vi "Create_filter_points.vi"(2 "Precision":string, 4 "Non-Blank Rows":bool[](array[boolean]), 6 "notSelectors?":bool, 7 "Index":i32, 8 "Channel to Filter On":i32, 9 "Tolerance":dbl=1.0 format="%.2f", 10 "Filter Bins 1":i32[](array[numeric]), 11 "Ch Values In":string[][](array[string])) -> (0 "Unchanged?":bool, 1 "Accept array":bool[][](array[boolean]), 3 "Filter Bins Out":i32[](array[numeric]), 5 "Bin Names":string[](array[string]))   [LabVIEW 2022 SP3]
uses:
  Results_plotter_Global.vi
panel:
  in  "Filter Info":T1={"Filter Bins"=[], "Channel to Filter On"=0, "Bin Matches"=[], "Number of Rows"=0, "Bin Names"=[], "Tolerance"=1.0, "Indicies for all bins"=[]} {"Tolerance" format="%.2f"}
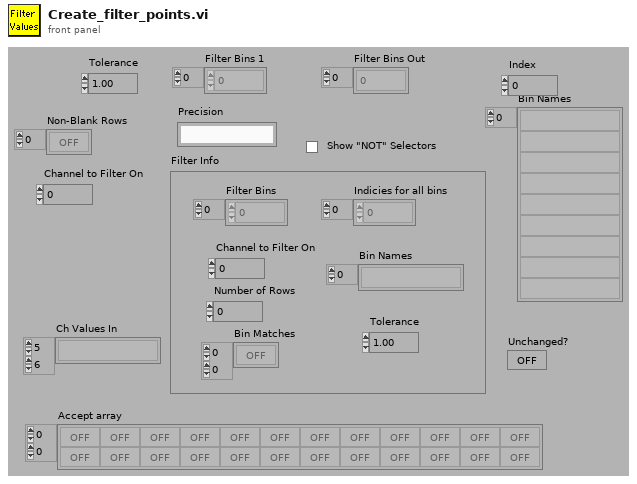
[diagram p1: front panel]
types:
  T1 = cluster{"Filter Bins":i32[], "Channel to Filter On":i32, "Bin Matches":bool[][], "Number of Rows":i32, "Bin Names":string[], "Tolerance":dbl, "Indicies for all bins":i32[]}
  T2 = cluster{"Filter Bins":i32[], "Channel to Filter On":i32, "Bin Matches":bool[][], "Number of Rows":i32, "Bin Names":string[], "Tolerance":dbl, "Indicies for all bins":i32[]}[]
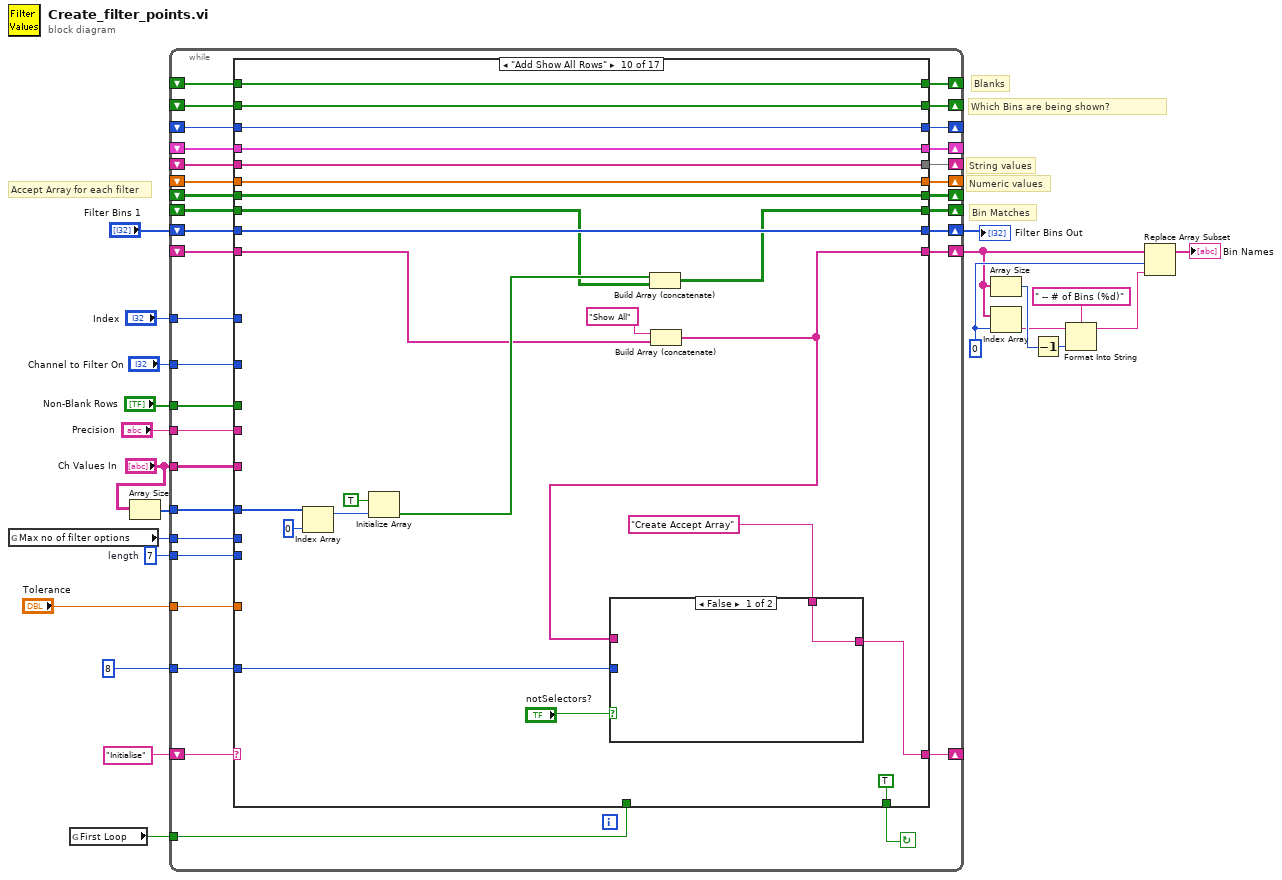
[diagram p0: block diagram]
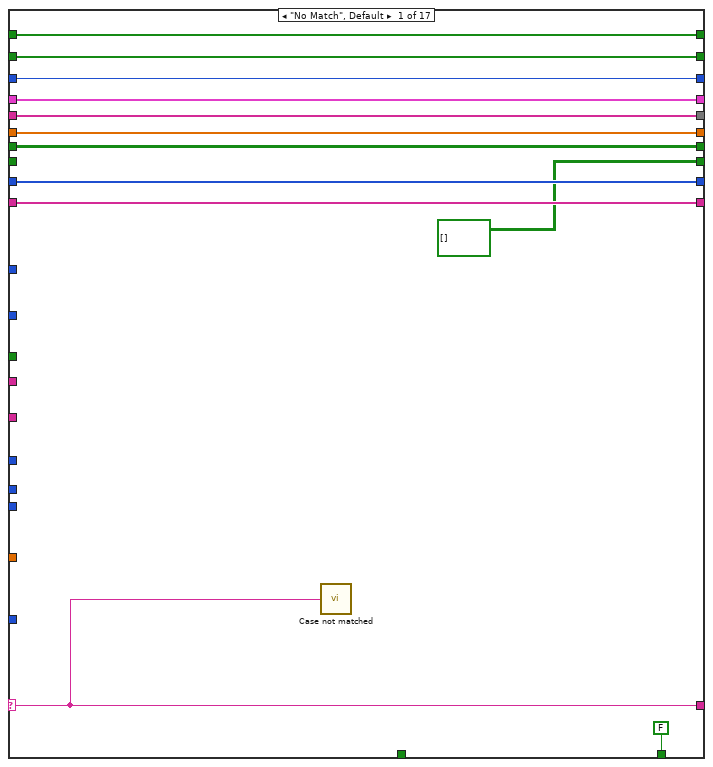
[diagram p2: hidden frame]
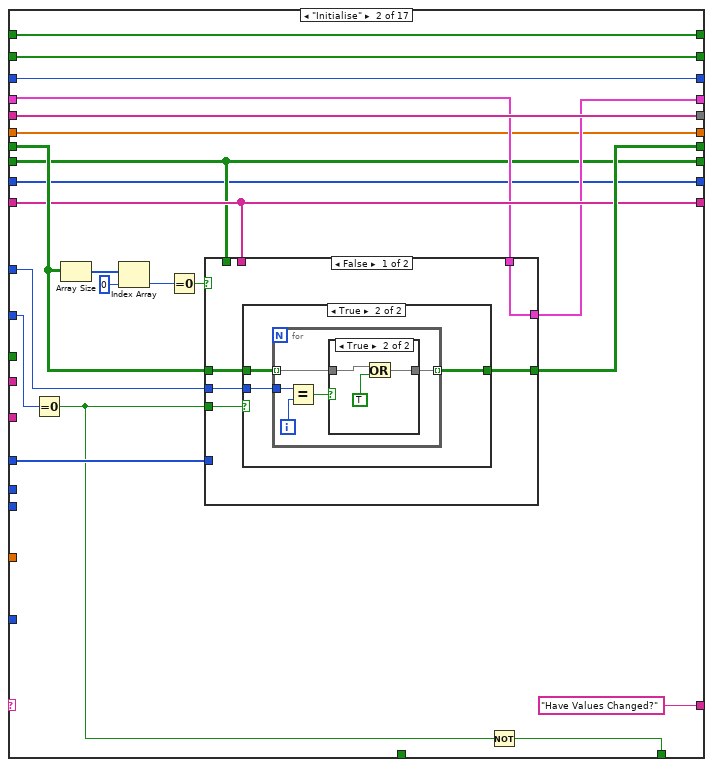
[diagram p3: hidden frame]
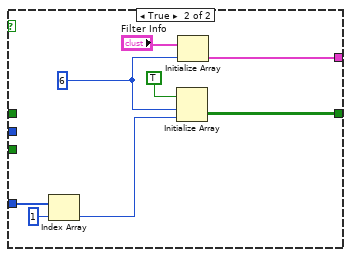
[diagram p6: hidden frame]
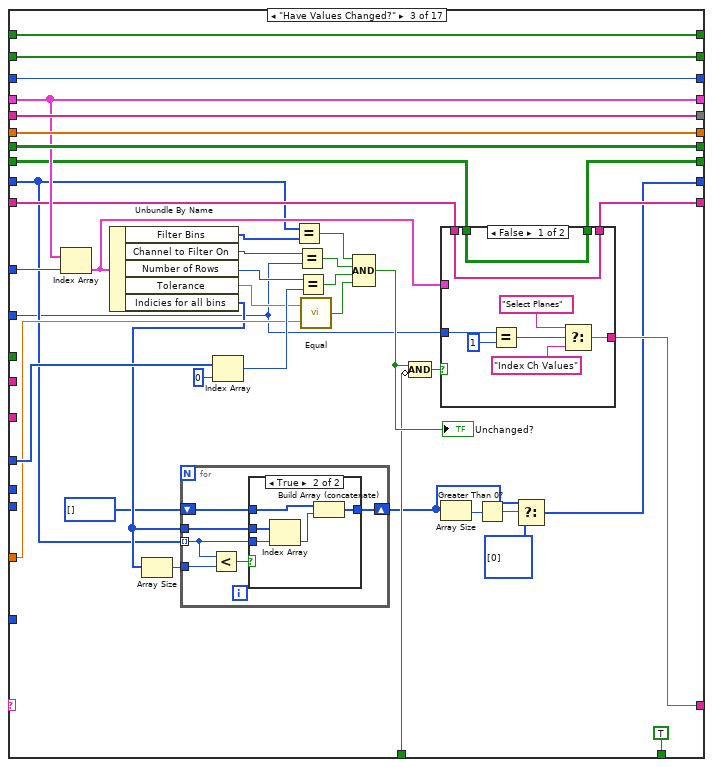
[diagram p7: hidden frame]
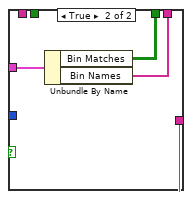
[diagram p9: hidden frame]
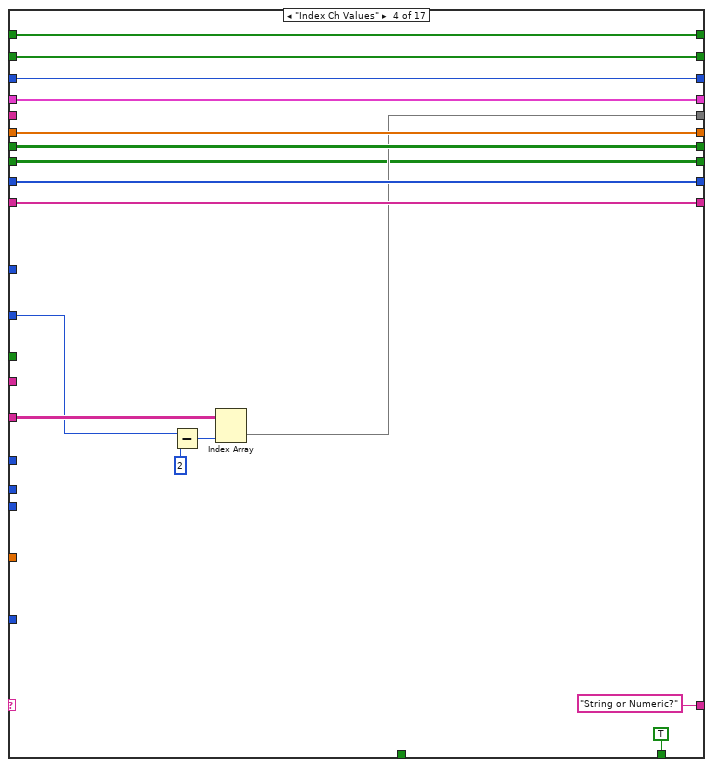
[diagram p10: hidden frame]
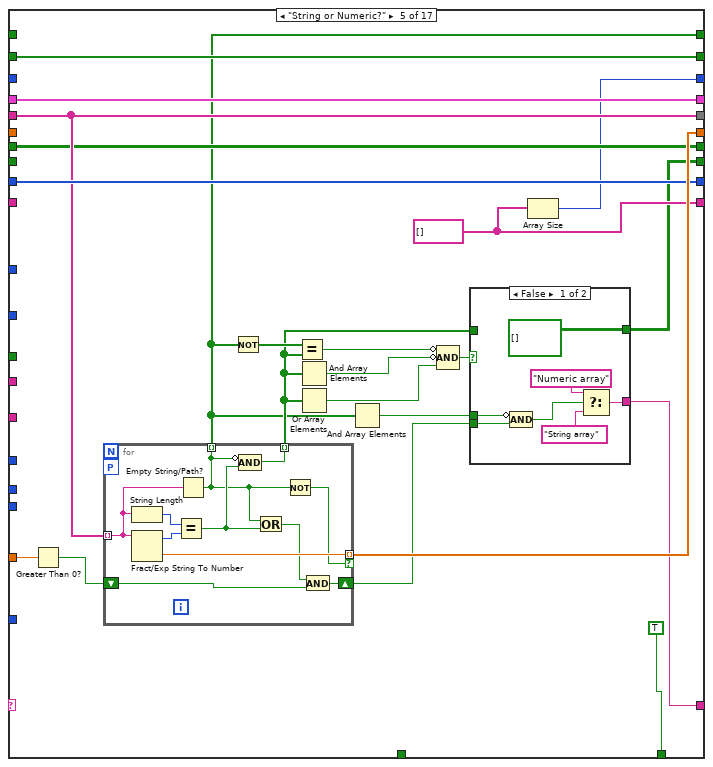
[diagram p11: hidden frame]
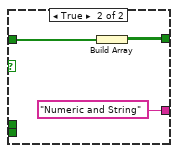
[diagram p12: hidden frame]
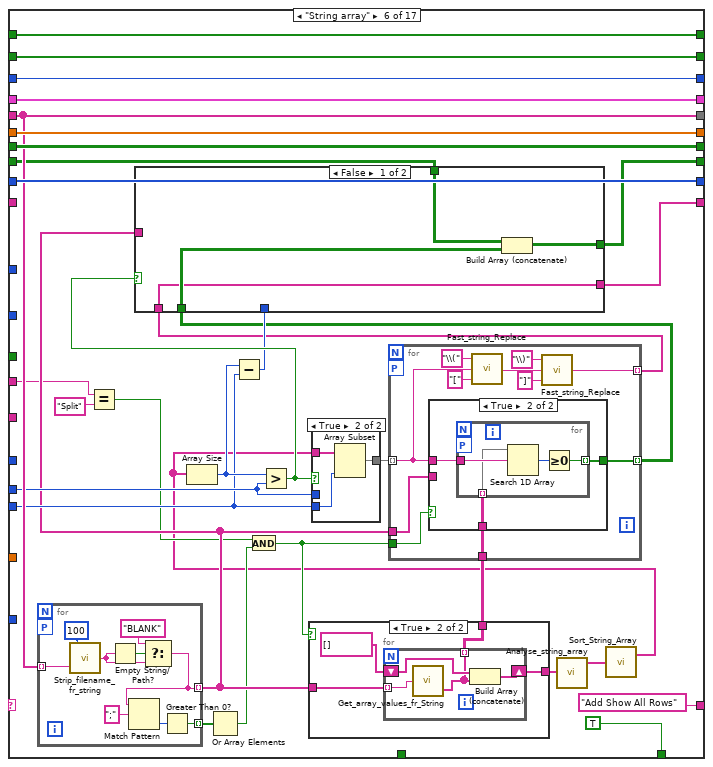
[diagram p13: hidden frame]
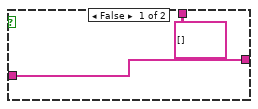
[diagram p14: hidden frame]
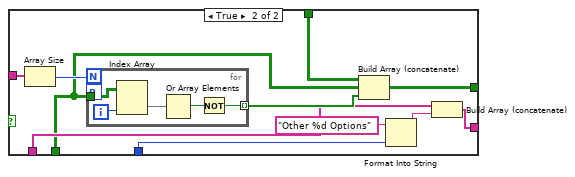
[diagram p15: hidden frame]
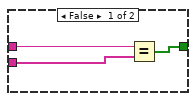
[diagram p17: hidden frame]
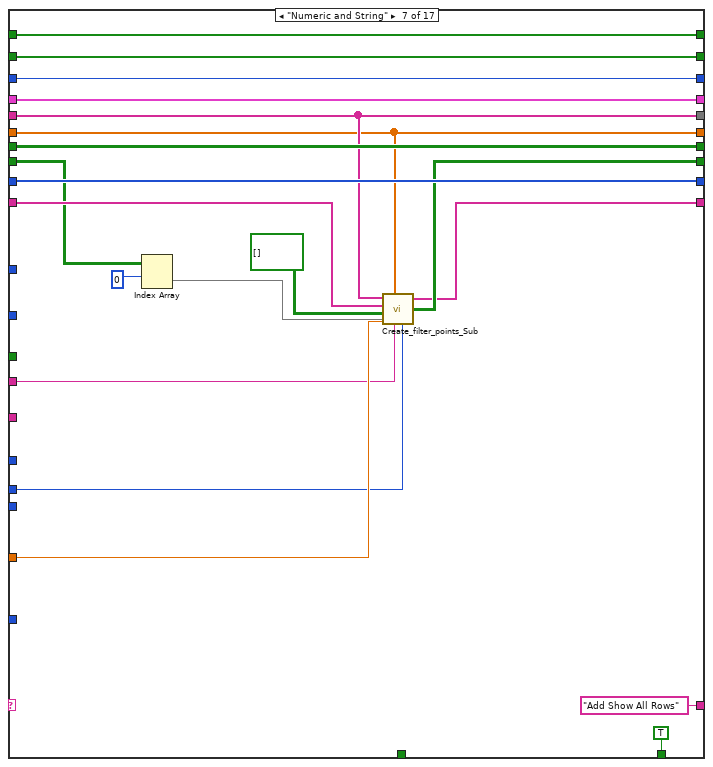
[diagram p18: hidden frame]
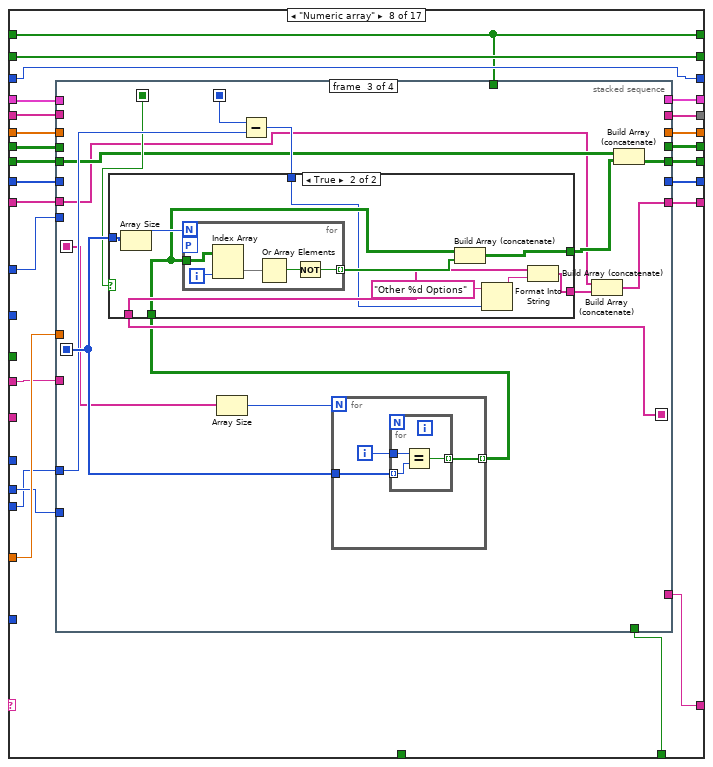
[diagram p19: hidden frame]
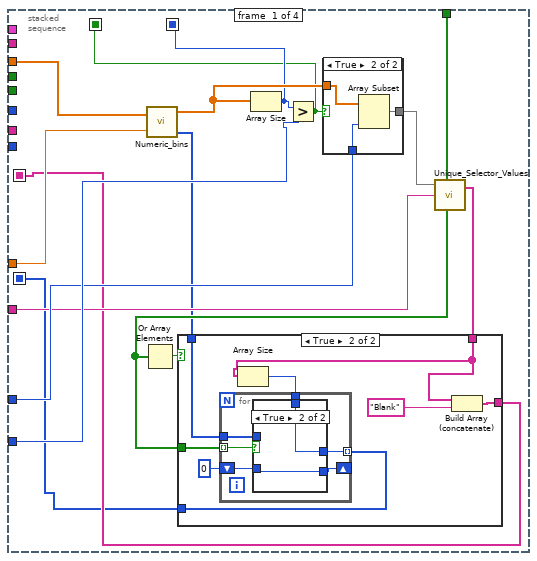
[diagram p20: hidden frame]
diagram:
  w7 = 0 ("index")
  w12 = 7  # length
  # "Blanks"
  # "Which Bins are being shown?"
  # "Accept Array for each filter"
  # "String values"
  # "Bin Matches"
  # "Numeric values"
  n1 = global read "Results_plotter_Global.vi" "Max no of filter options"() -> (w13:i32)
  n2 = global read "Results_plotter_Global.vi" "First Loop"() -> (w16:bool)
  n3 = Array Size(array="Ch Values In") -> (size(s)=w18:i32[])
  n4 = while {
    tunnel: "Non-Blank Rows" -> [w38]
    tunnel: w18 -> [w39]
    tunnel: "Channel to Filter On" -> [w41]
    shift-left: _ -> [w43]
    shift-right: [w42] -> _
    shift-left: _ -> [w44]
    shift-right: [w40] -> _
    shift-left: "Filter Bins 1" -> [w46]
    shift-right: [w45] -> w10
    tunnel: "Index" -> [w48]
    shift-left: _ -> [w47]
    shift-right: [w49] -> w6
    shift-left: _ -> [w35]
    shift-right: [w32] -> _
    shift-left: _ -> [w53]
    shift-right: [w52] -> _
    shift-left: _ -> [w50]
    shift-right: [w55] -> _
    shift-left: "Initialise" -> [w51]
    shift-right: [w25] -> _
    tunnel: "Ch Values In" -> [w56]
    tunnel: w16 -> [w37]
    tunnel: "Tolerance" -> [w36]
    shift-right: [w34] -> _
    shift-left: _ -> [w33]
    tunnel: "Precision" -> [w31]
    shift-right: [w30] -> _
    shift-left: _ -> [w29]
    tunnel: w13 -> [w28]
    tunnel: w12 -> [w27]
    tunnel: 8 ("y") -> [w26]
    shift-right: [w24] -> _
    shift-left: _ -> [w23]
    stop <- w54 continue-if-true
    n5 = case shown="\"Add Show All Rows\"" w51 {
      selector: w51 -> [w57 _ _ _ _ _ _ _ _ _ _ _ _ _ _ _ _]
      tunnel: w56 -> [_ _ _ w188 _ _ _ _ w501 _ _ _ _ _ _ _ _]
      tunnel: [w67 w76 w155 w194 w218 w270 w343 w376 w521 w704 w731 w752 w795 w848 w867 w895 w935] -> w55
      tunnel: [w57 "Have Values Changed?" w140 "String or Numeric?" w204 "Add Show All Rows" "Add Show All Rows" w378 w523 w689 "Create Accept Array" "Add Number of hits" "Relocate Selector?" w837 "Stop invalid selections" "Update shift Register" "End"] -> w25
      tunnel: [FALSE w79 TRUE TRUE TRUE TRUE TRUE w379 w524 TRUE TRUE TRUE TRUE TRUE TRUE TRUE FALSE] -> w54
      tunnel: w53 -> [w66 w86 w154 w193 w212 w267 w352 w374 w519 w703 w730 w747 w792 w846 w866 w894 w934]
      tunnel: [w66 w87 w154 w193 w212 w267 w352 w373 w518 w703 w730 w746 w792 w846 w866 w894 w934] -> w52
      tunnel: w50 -> [w67 w76 w155 w194 _ w270 w343 w375 w520 w704 w731 w752 w795 w848 w867 w895 w935]
      tunnel: [w65 w82 w139 w191 w200 w257 w344 w377 w522 w691 w718 w750 w790 w845 w864 w892 w914] -> w49
      tunnel: w48 -> [_ w85 w152 _ _ _ _ w369 w514 _ _ w749 w796 w835 w863 _ w932]
      tunnel: w35 -> [_ w77 w141 w187 _ w260 w346 w371 w516 w697 w723 w740 w784 w847 w859 w890 w925]
      tunnel: w47 -> [w65 w82 w138 w191 _ _ w347 w363 w508 w696 w719 w750 w787 w845 w864 w892 w917]
      tunnel: w46 -> [w62 w75 w119 w192 w216 w266 w351 w370 w515 w707 w734 w744 w799 w850 w857 w888 w912]
      tunnel: [w62 w75 w120 w192 w216 w266 w351 w364 w509 w707 w734 w744 w799 w850 w852 w884 w911] -> w45
      tunnel: w44 -> [w64 w84 w153 _ w214 w264 w350 w368 w513 w705 w732 w753 w797 w849 w865 w893 w933]
      tunnel: w43 -> [w63 w80 w151 w190 w215 w268 w353 w366 w511 w706 w733 w754 w798 w843 w855 w887 w931]
      tunnel: [w63 w81 w151 w190 w215 w268 w353 w365 w510 w706 w733 w754 w798 w843 w855 w887 w930] -> w42
      tunnel: w41 -> [_ w83 w118 w183 _ _ _ _ _ _ _ _ _ _ _ _ w924]
      tunnel: [w64 w84 w153 w189 w214 w264 w350 w367 w512 w705 w732 w753 w797 w849 w865 w893 w933] -> w40
      tunnel: [bool[][] [] w77 w128 w187 w199 w258 w345 w372 w517 w688 w722 w740 w784 w847 w859 w890 w925] -> w32
      tunnel: w39 -> [_ w74 w150 _ _ _ _ _ _ w701 _ _ _ _ _ _ w929]
      tunnel: w38 -> [_ _ _ _ _ _ _ _ _ _ _ w743 w794 _ _ _ _]
      tunnel: w37 -> [_ _ w132 _ _ _ _ _ _ _ _ _ _ _ _ _ _]
      tunnel: w36 -> [_ _ w131 _ w203 _ w349 w362 w507 _ _ _ _ _ _ _ w920]
      tunnel: [w61 w71 w130 w186 w202 w265 w342 w357 w502 w693 w727 w742 w791 w834 w854 w886 w919] -> w34
      tunnel: w33 -> [w61 w71 w130 w186 _ w265 w342 w357 w502 w693 w727 w742 w791 w834 w854 w886 w919]
      tunnel: w31 -> [_ _ _ _ _ w246 w341 w361 w506 _ _ _ _ _ _ _ _]
      tunnel: [w59 w70 w129 w185 w201 w263 w340 w360 w505 w692 w717 w741 w789 w833 w853 w885 w918] -> w30
      tunnel: w29 -> [w59 w70 w129 w185 w201 w263 w340 w360 w505 w692 w717 w741 _ w833 w853 w885 w918]
      tunnel: w28 -> [_ _ _ _ _ w261 w339 w359 w504 _ _ _ w776 _ _ _ _]
      tunnel: w27 -> [_ _ _ _ _ w255 _ w358 w503 _ _ _ _ _ _ _ _]
      tunnel: w26 -> [_ _ _ _ _ _ _ _ _ w687 _ _ w778 _ _ _ _]
      tunnel: [w58 w69 w117 w181 w197 w240 w336 w356 w498 w686 w716 w739 w775 w832 w851 w883 w910] -> w24
      tunnel: w23 -> [w58 w69 w117 w181 _ w240 w336 w356 w498 w686 w716 w739 w775 w832 w851 w883 w910]
      frame "No Match", Default {
        n6 = call "Case not matched.vi"("Case Name not Matched"=w57) -> ()
      }
      frame "Initialise" {
        n7 = Equal To 0?(x=w83) -> (x = 0?=w73:bool)
        n8 = Array Size(array=w86) -> (size(s)=w90:i32[])
        n9 = Index Array(array=w90, index=0 ("Index")) -> (element=w88:i32)
        n10 = Equal To 0?(x=w88) -> (x = 0?=w72:bool)
        n11 = case shown="False" w72 {
          tunnel: [w95 w115] -> w87
          tunnel: w86 -> [w94 _]
          tunnel: w85 -> [w93 _]
          tunnel: w73 -> [w92 _]
          tunnel: w82 -> [_ _]
          tunnel: [w91 w113] -> w81
          tunnel: w80 -> [w91 _]
          tunnel: w77 -> [_ _]
          tunnel: w74 -> [_ w110]
          frame False {
            n12 = case shown="True" w92 {
              tunnel: [w96 w98] -> w95
              tunnel: w94 -> [w96 w97]
              tunnel: w93 -> [_ w99]
              frame False {
              }
              frame True {
                n13 = for {
                  tunnel: w99 -> [w104]
                  tunnel: [w101] -> w98 mode=indexing
                  tunnel: w97 -> [w100] mode=indexing
                  i -> [w103]
                  n14 = Equal?(x=w104, y=w103) -> (x = y?=w102:bool)
                  n15 = case shown="True" w102 {
                    tunnel: [w105 w106] -> w101
                    tunnel: w100 -> [w105 w107]
                    frame False {
                    }
                    frame True {
                      n16 = Or(x=w107, y=TRUE) -> (x .or. y?=w106:bool[])
                    }
                  }
                }
              }
            }
          }
          frame True {
            w114 = 6 ("Dimension Size")
            n17 = Index Array(array=w110, index=1 ("Index")) -> (element=w111:i32)
            n18 = Initialize Array(TRUE, w114, w111) -> (w115:bool[][])
            n19 = Initialize Array("Filter Info", w114) -> (w113:T2)
          }
        }
        n20 = Not(x=w73) -> (.not. x?=w79:bool)
      }
      frame "Have Values Changed?" {
        n21 = Index Array(array=w151, index=w152) -> (element=w142:T1)
        n22 = Unbundle By Name(w142) -> ("Filter Bins"=w137:i32[], "Channel to Filter On"=w148:i32, "Number of Rows"=w147:i32, "Tolerance"=w134:dbl, "Indicies for all bins"=w127:i32[])
        n23 = Array Size(array=w127) -> (size(s)=w126:i32)
        n24 = for {
          tunnel: w119 -> [w160] mode=indexing
          tunnel: w127 -> [w162]
          tunnel: w126 -> [w161]
          shift-right: [w158] -> w122
          shift-left: i32[] [] -> [w157]
          n25 = Less?(x=w160, y=w161) -> (x < y?=w159:bool)
          n26 = case shown="True" w159 {
            tunnel: w162 -> [_ w168]
            tunnel: w160 -> [_ w167]
            tunnel: [w163 w165] -> w158
            tunnel: w157 -> [w163 w164]
            frame False {
            }
            frame True {
              n27 = Index Array(array=w168, index=w167) -> (element=w166:i32)
              n28 = Build Array (concatenate)(w164, w166) -> (w165:i32[])
            }
          }
        }
        n29 = Index Array(array=w150, index=0 ("Index")) -> (element=w146:i32)
        n30 = Equal?(x=w119, y=w137) -> (x = y?=w145:bool)
        n31 = Equal?(x=w148, y=w118) -> (x = y?=w144:bool)
        n32 = Equal?(x=w147, y=w146) -> (x = y?=w143:bool)
        n33 = call "Equal.vi"("Input2"=w131, "Input1"=w134) -> ("Equal?"=w133:bool)
        n34 = Compound Arithmetic op=AND(w145, w144, w143, w133) -> (w135:bool)
        "Unchanged?" <- w135
        n35 = Compound Arithmetic op=AND(w135, invert w132) -> (w136:bool)
        n36 = case shown="False" w136 {
          tunnel: w142 -> [_ w180]
          tunnel: [w175 w178] -> w128
          tunnel: w141 -> [w175 _]
          tunnel: [w170 "Create Accept Array"] -> w140
          tunnel: [w176 w179] -> w139
          tunnel: w138 -> [w176 _]
          tunnel: w118 -> [w174 _]
          frame False {
            n37 = Equal?(x=w174, y=1) -> (x = y?=w172:bool)
            n38 = Select(t="Select Planes", s=w172, f="Index Ch Values") -> (s? t:f=w170:string)
          }
          frame True {
            n39 = Unbundle By Name(w180) -> ("Bin Matches"=w178:bool[][], "Bin Names"=w179:string[])
          }
        }
        n40 = Array Size(array=w122) -> (size(s)=w124:i32)
        n41 = Greater Than 0?(x=w124) -> (x > 0?=w123:bool)
        n42 = Select(t=w122, s=w123, f=i32[] [0]) -> (s? t:f=w120:i32[])
      }
      frame "Index Ch Values" {
        n43 = Subtract(x=w183, y=2) -> (x-y=w182:i32)
        n44 = Index Array(array=w188, index (col)=w182) -> (element=w189:string[])  [unwired: 1 in]
      }
      frame "String or Numeric?" {
        w200 = string[] []
        n45 = Greater Than 0?(x=w203) -> (x > 0?=w217:bool)
        n46 = for {
          tunnel: w214 -> [w235] mode=indexing
          shift-right: [w238] -> w205
          shift-left: w217 -> [w239]
          tunnel: [w232] -> w218 mode=indexing if=w230
          tunnel: [w229] -> w197 mode=indexing
          tunnel: [w233] -> w198 mode=indexing
          workers-P: _ -> [_]
          n47 = String Length(string=w235) -> (length=w236:i32)
          n48 = Fract/Exp String To Number(string=w235) -> (offset past number=w237:i32, number=w232:dbl)  [unwired: 3 out]
          n49 = Equal?(x=w236, y=w237) -> (x = y?=w234:bool)
          n50 = Empty String/Path?(string/path=w235) -> (empty?=w229:bool)
          n51 = Compound Arithmetic op=AND(invert w229, w234) -> (w233:bool)
          n52 = Or(x=w229, y=w234) -> (x .or. y?=w231:bool)
          n53 = Not(x=w229) -> (.not. x?=w230:bool)
          n54 = And(x=w231, y=w239) -> (x .and. y?=w238:bool)
        }
        n55 = Not(x=w197) -> (.not. x?=w207:bool[])
        n56 = Equal?(x=w207, y=w198) -> (x = y?=w208:bool)
        n57 = And Array Elements(Boolean array=w198) -> (logical AND=w211:bool)
        n58 = Or Array Elements(Boolean array=w198) -> (logical OR=w210:bool)
        n59 = And Array Elements(Boolean array=w197) -> (logical AND=w206:bool)
        n60 = Compound Arithmetic op=AND(invert w208, invert w211, w210) -> (w209:bool)
        n61 = case shown="False" w209 {
          tunnel: w206 -> [w225 _]
          tunnel: w205 -> [w224 _]
          tunnel: [w220 "Numeric and String"] -> w204
          tunnel: [bool[][] [] w226] -> w199
          tunnel: w198 -> [_ w227]
          frame False {
            n62 = Compound Arithmetic op=AND(invert w225, w224) -> (w221:bool)
            n63 = Select(t="Numeric array", s=w221, f="String array") -> (s? t:f=w220:string)
          }
          frame True {
            n64 = Build Array(w227) -> (w226:bool[][])
          }
        }
        n65 = Array Size(array=w200) -> (size(s)=w202:i32)
      }
      frame "String array" {
        n66 = for {
          tunnel: w264 -> [w314] mode=indexing
          tunnel: [w306] -> w249 mode=indexing
          tunnel: [w310] -> w251 mode=indexing
          workers-P: _ -> [_]
          n67 = call "Strip_filename_fr_string.vi"("Input String"=w314, "y"=100) -> ("Output String"=w307:string)
          n68 = Empty String/Path?(string/path=w307) -> (empty?=w309:bool)
          n69 = Select(t="BLANK", s=w309, f=w307) -> (s? t:f=w306:string)
          n70 = Match Pattern(string=w306, regular expression=";") -> (offset past match=w311:i32)  [unwired: 4 out]
          n71 = Greater Than 0?(x=w311) -> (x > 0?=w310:bool)
        }
        n72 = Equal?(x=w246, y="Split") -> (x = y?=w244:bool)
        n73 = Or Array Elements(Boolean array=w251) -> (logical OR=w245:bool)
        n74 = And(x=w244, y=w245) -> (x .and. y?=w243:bool)
        n75 = case shown="True" w243 {
          tunnel: [w273 w276] -> w250
          tunnel: w249 -> [w273 w275]
          tunnel: [string[][] [] ("String array") w274] -> w248
          frame False {
          }
          frame True {
            n76 = for {
              shift-right: [w281] -> w276
              shift-left: string[] [] -> [w280]
              tunnel: w275 -> [w279] mode=indexing
              tunnel: [w278] -> w274 mode=indexing
              n77 = call "Get_array_values_fr_String.vi"("String Value"=w279) -> ("String array"=w278:string[])  [unwired: 1 out]
              n78 = Build Array (concatenate)(w280, w278) -> (w281:string[])
            }
          }
        }
        n79 = call "Analyse_string_array.vi"("String array"=w250) -> ("Unique strings"=w242:string[])  [unwired: 2 out]
        n80 = call "Sort_String_Array.vi"("Unsorted String"=w242) -> ("Sorted String"=w241:string[])  [unwired: 1 out]
        n81 = Array Size(array=w241) -> (size(s)=w256:i32)
        n82 = Subtract(x=w256, y=w255) -> (x-y=w254:i32)
        n83 = Greater?(x=w256, y=w261) -> (0:w259:bool)
        n84 = case shown="True" w259 {
          tunnel: w241 -> [w302 w305]
          tunnel: w261 -> [_ _]
          tunnel: [w302 w304] -> w262
          tunnel: w255 -> [_ w303]
          frame False {
          }
          frame True {
            n85 = Array Subset(array=w305, length=w303) -> (w304:string[])  [unwired: 1 in]
          }
        }
        n86 = for {
          tunnel: w249 -> [w320]
          tunnel: w262 -> [w319] mode=indexing
          tunnel: [w315] -> w253 mode=indexing
          tunnel: [w318] -> w252 mode=indexing
          tunnel: w243 -> [w317]
          tunnel: w248 -> [w316]
          workers-P: _ -> [_]
          n87 = case shown="True" w317 {
            tunnel: w320 -> [w328 _]
            tunnel: w319 -> [w327 w331]
            tunnel: [w326 w330] -> w318
            tunnel: w316 -> [_ w329]
            frame False {
              n88 = Equal?(x=w327, y=w328) -> (x = y?=w326:bool[])
            }
            frame True {
              n89 = for {
                tunnel: w331 -> [w335]
                tunnel: [w333] -> w330 mode=indexing
                tunnel: w329 -> [w332] mode=indexing
                workers-P: _ -> [_]
                n90 = Search 1D Array(1D array=w332, element=w335) -> (index of element=w334:i32)  [unwired: 1 out]
                n91 = Greater Or Equal To 0?(x=w334) -> (x >= 0?=w333:bool)
              }
            }
          }
          n92 = call "Fast_string_Replace.vi"("Replace match with:"="[", "Input String"=w319, "regular expression"="\\(") -> ("Output String"=w321:string)  [unwired: 2 out]
          n93 = call "Fast_string_Replace.vi"("Replace match with:"="]", "Input String"=w321, "regular expression"="\\)") -> ("Output String"=w315:string)  [unwired: 2 out]
        }
        n94 = case shown="False" w259 {
          tunnel: w253 -> [w283 w293]
          tunnel: w260 -> [w285 w296]
          tunnel: w252 -> [w284 w286]
          tunnel: [w282 w294] -> w258
          tunnel: [w283 w292] -> w257
          tunnel: w249 -> [_ w291]
          tunnel: w254 -> [_ w289]
          frame False {
            n95 = Build Array (concatenate)(w285, w284) -> (w282:bool[][])
          }
          frame True {
            n96 = Array Size(array=w291) -> (size(s)=w290:i32)
            n97 = for {
              N: w290 -> [_]
              tunnel: w286 -> [w301]
              tunnel: [w297] -> w295 mode=indexing
              workers-P: _ -> [_]
              i -> [w300]
              n98 = Index Array(array=w301, index (col)=w300) -> (element=w299:bool[])  [unwired: 1 in]
              n99 = Or Array Elements(Boolean array=w299) -> (logical OR=w298:bool)
              n100 = Not(x=w298) -> (.not. x?=w297:bool)
            }
            n101 = Build Array (concatenate)(w296, w286, w295) -> (w294:bool[][])
            n102 = Format Into String(format string="Other %d Options", w289) -> (resulting string=w287:string)  [unwired: 2 in, 1 out]
            n103 = Build Array (concatenate)(w293, w287) -> (w292:string[])
          }
        }
      }
      frame "Numeric and String" {
        n104 = Index Array(array=w346, index (row)=0) -> (element=w348:bool[])  [unwired: 1 in]
        n105 = call "Create_filter_points_Sub.vi"("Numeric Value?"=w348, "No of filter options"=w339, "Precision"=w341, "Tolerance"=w349, "Bin Matches in"=bool[][] [] ("Bin Matches"), "Numeric Array"=w343, "Bin Names In"=w347, "String Array"=w350) -> ("Bin Matches"=w345:bool[][], "Bin Names"=w344:string[])  [unwired: 1 out]
      }
      frame "Numeric array" {
        n106 = stacked-sequence {
          seq-local: [w381 _ _ _] -> [_ _ w466 _]
          seq-local: [_ w422 _ _] -> [_ _ w467 _]
          seq-local: [w389 _ _ _] -> [_ _ w465 _]
          seq-local: [w388 _ _ _] -> [_ _ w462 _]
          seq-local: [w383 _ _ _] -> [_ w421 w453 _]
          tunnel: w362 -> [w393 _ _ _]
          tunnel: [_ _ _ w493] -> w376
          tunnel: w375 -> [w394 _ _ w493]
          tunnel: w374 -> [_ _ _ w492]
          tunnel: [_ _ _ w492] -> w373
          tunnel: [_ _ w459 _] -> w372
          tunnel: w371 -> [_ _ w458 _]
          tunnel: w370 -> [_ _ _ w491]
          tunnel: [_ _ _ w491] -> w364
          tunnel: [_ _ _ TRUE] -> w379
          tunnel: [_ _ _ "Add Show All Rows"] -> w378
          tunnel: [_ _ w456 _] -> w377
          tunnel: w369 -> [_ _ _ _]
          tunnel: w368 -> [_ _ _ w495]
          tunnel: [_ _ _ w495] -> w367
          tunnel: w366 -> [_ _ _ w494]
          tunnel: [_ _ _ w494] -> w365
          tunnel: w363 -> [_ _ w455 _]
          tunnel: w361 -> [w386 _ _ _]
          tunnel: w359 -> [w391 _ _ _]
          tunnel: w358 -> [w390 _ w464 _]
          tunnel: w356 -> [w382 _ _ _]
          frame #0 {
            n107 = Or Array Elements(Boolean array=w382) -> (logical OR=w385:bool)
            n108 = call "Numeric_bins.vi"("Values"=w394, "Tolerance"=w393) -> ("Bin Centres"=w392:dbl[], "Bin Index"=w380:i32[])  [unwired: 1 out]
            n109 = Array Size(array=w392) -> (size(s)=w389:i32)
            n110 = Greater?(x=w389, y=w391) -> (0:w388:bool)
            n111 = case shown="True" w388 {
              tunnel: w392 -> [w417 w420]
              tunnel: [w417 w419] -> w387
              tunnel: w390 -> [_ w418]
              frame False {
              }
              frame True {
                n112 = Array Subset(array=w420, length=w418) -> (w419:dbl[])  [unwired: 1 in]
              }
            }
            n113 = call "Unique_Selector_Values.vi"("Precision"=w386, "Bin Centres"=w387) -> ("Bin Strings"=w384:string[])  [unwired: 1 in, 1 out]
            n114 = case shown="True" w385 {
              tunnel: w384 -> [w396 w402]
              tunnel: [w396 w403] -> w383
              tunnel: w382 -> [_ w401]
              tunnel: [w395 w400] -> w381
              tunnel: w380 -> [w395 w397]
              frame False {
              }
              frame True {
                n115 = Array Size(array=w402) -> (size(s)=w399:i32)
                n116 = for {
                  shift-right: [w406] -> _
                  shift-left: 0 -> [w407]
                  tunnel: w401 -> [w410] mode=indexing
                  tunnel: [w409] -> w400 mode=indexing
                  tunnel: w399 -> [w408]
                  tunnel: w397 -> [w405]
                  n117 = case shown="True" w410 {
                    tunnel: [w412 w416] -> w409
                    tunnel: w408 -> [_ w416]
                    tunnel: w407 -> [w414 w415]
                    tunnel: [w413 w415] -> w406
                    tunnel: w405 -> [w411 _]
                    frame False {
                      n118 = Index Array(array=w411, index=w414) -> (element=w412:i32)
                      n119 = Increment(x=w414) -> (x+1=w413:i32)
                    }
                    frame True {
                    }
                  }
                }
                n120 = Build Array (concatenate)(w402, "Blank" ("String")) -> (w403:string[])
              }
            }
          }
          frame #1 {
            n121 = for {
              tunnel: [w424] -> w422 mode=indexing
              tunnel: w421 -> [w423] mode=indexing
              workers-P: _ -> [_]
              n122 = Match Pattern(string=w423, regular expression="[.]") -> (offset past match=w425:i32)  [unwired: 4 out]
              n123 = case shown="0, Default" w425 {
                tunnel: [w434 w452] -> w424
                tunnel: w423 -> [w436 w452]
                frame 0, Default {
                  n124 = Reverse String(1:w436) -> (0:w435:string)
                  n125 = while {
                    shift-right: [w442] -> w429
                    shift-left: w435 -> [w443]
                    stop <- w441 continue-if-true
                    n126 = String Subset(string=w443, offset (0)=0, length (rest)=1 ("length (rest)")) -> (substring=w445:string)
                    n127 = Equal?(x=w445, y="0") -> (x = y?=w441:bool)
                    n128 = case shown="False" w441 {
                      tunnel: w443 -> [w448 w450]
                      tunnel: [w448 w449] -> w442
                      frame False {
                      }
                      frame True {
                        n129 = String Subset(string=w450, offset (0)=1) -> (substring=w449:string)  [unwired: 1 out]
                      }
                    }
                  }
                  n130 = String Subset(string=w429, offset (0)=0, length (rest)=1 ("length (rest)")) -> (substring=w431:string)
                  n131 = Equal?(x=w431, y=".") -> (x = y?=w428:bool)
                  n132 = case shown="False" w428 {
                    tunnel: w429 -> [w437 w439]
                    tunnel: [w437 w438] -> w427
                    frame False {
                    }
                    frame True {
                      n133 = String Subset(string=w439, offset (0)=1) -> (substring=w438:string)  [unwired: 1 out]
                    }
                  }
                  n134 = Reverse String(1:w427) -> (0:w434:string)
                }
                frame -1 {
                }
              }
            }
          }
          frame #2 {
            n135 = Array Size(array=w453) -> (size(s)=w454:i32)
            n136 = Subtract(x=w465, y=w464) -> (x-y=w463:i32)
            n137 = for {
              N: w454 -> [_]
              tunnel: w466 -> [w487]
              tunnel: [w486] -> w460 mode=indexing
              i -> [w485]
              n138 = for {
                tunnel: w487 -> [w490] mode=indexing
                tunnel: w485 -> [w489]
                tunnel: [w488] -> w486 mode=indexing
                n139 = Equal?(x=w489, y=w490) -> (x = y?=w488:bool)
              }
            }
            n140 = case shown="True" w462 {
              tunnel: w467 -> [w469 w477]
              tunnel: w460 -> [w468 w471]
              tunnel: [w468 w478] -> w461
              tunnel: [w469 w476] -> w457
              tunnel: w466 -> [_ w475]
              tunnel: w463 -> [_ w470]
              frame False {
              }
              frame True {
                n141 = Array Size(array=w475) -> (size(s)=w474:i32)
                n142 = for {
                  N: w474 -> [_]
                  tunnel: w471 -> [w484]
                  tunnel: [w480] -> w479 mode=indexing
                  workers-P: _ -> [_]
                  i -> [w483]
                  n143 = Index Array(array=w484, index (col)=w483) -> (element=w482:bool[])  [unwired: 1 in]
                  n144 = Or Array Elements(Boolean array=w482) -> (logical OR=w481:bool)
                  n145 = Not(x=w481) -> (.not. x?=w480:bool)
                }
                n146 = Build Array (concatenate)(w471, w479) -> (w478:bool[][])
                n147 = Format Into String(format string="Other %d Options", w470) -> (resulting string=w472:string)  [unwired: 2 in, 1 out]
                n148 = Build Array (concatenate)(w477, w472) -> (w476:string[])
              }
            }
            n149 = Build Array (concatenate)(w455, w457) -> (w456:string[])
            n150 = Build Array (concatenate)(w458, w461) -> (w459:bool[][])
          }
          frame #3 {
          }
        }
      }
      frame "Select Planes" {
        n151 = global read "Results_plotter_Global.vi" "3D Ch Selectors"() -> (w500:i32[])
        n152 = global read "Results_plotter_Global.vi" "Precision"() -> (w499:string[])
        n153 = stacked-sequence {
          seq-local: [w538 _ _ _ _ _] -> [_ w596 _ _ _ _]
          seq-local: [w537 _ _ _ _ _] -> [_ w598 _ _ _ _]
          seq-local: [w536 _ _ _ _ _] -> [_ w586 _ _ _ _]
          seq-local: [w535 _ _ _ _ _] -> [_ w599 w627 w655 _ _]
          seq-local: [_ w588 _ _ _ _] -> [_ _ _ _ w677 _]
          seq-local: [_ w587 _ _ _ _] -> [_ _ _ _ w672 _]
          seq-local: [w533 _ _ _ _ _] -> [_ _ w616 _ _ _]
          seq-local: [w532 _ _ _ _ _] -> [_ _ w615 _ _ _]
          seq-local: [w531 _ _ _ _ _] -> [_ _ w614 _ _ _]
          seq-local: [w530 _ _ _ _ _] -> [_ _ _ w642 _ _]
          seq-local: [w529 _ _ _ _ _] -> [_ _ _ w643 _ _]
          seq-local: [w528 _ _ _ _ _] -> [_ _ _ w644 _ _]
          seq-local: [_ _ w618 _ _ _] -> [_ _ _ _ w676 _]
          seq-local: [_ _ w617 _ _ _] -> [_ _ _ _ w671 _]
          seq-local: [_ _ _ w646 _ _] -> [_ _ _ _ w670 _]
          seq-local: [_ _ _ w645 _ _] -> [_ _ _ _ w675 _]
          tunnel: w507 -> [_ _ _ _ _ _]
          tunnel: [_ _ _ _ _ w680] -> w521
          tunnel: w520 -> [_ _ _ _ _ w680]
          tunnel: w519 -> [_ _ _ _ _ w679]
          tunnel: [_ _ _ _ _ w679] -> w518
          tunnel: [_ _ _ _ w674 _] -> w517
          tunnel: w516 -> [_ _ _ _ _ _]
          tunnel: w515 -> [_ _ _ _ _ w678]
          tunnel: [_ _ _ _ _ w678] -> w509
          tunnel: [_ _ _ _ _ TRUE] -> w524
          tunnel: [_ _ _ _ _ "Add Show All Rows"] -> w523
          tunnel: [_ _ _ _ w673 _] -> w522
          tunnel: w514 -> [_ _ _ _ _ _]
          tunnel: w513 -> [_ _ _ _ _ w682]
          tunnel: [_ _ _ _ _ w682] -> w512
          tunnel: w511 -> [_ _ _ _ _ w681]
          tunnel: [_ _ _ _ _ w681] -> w510
          tunnel: w508 -> [_ _ _ _ _ _]
          tunnel: w506 -> [_ _ _ _ _ _]
          tunnel: w504 -> [_ _ _ _ _ _]
          tunnel: w503 -> [_ _ _ _ _ _]
          tunnel: w501 -> [w547 _ _ _ _ _]
          tunnel: w500 -> [w534 w594 w624 w652 _ _]
          tunnel: w499 -> [_ w593 w623 w651 _ _]
          frame #0 {
            w539 = 5 ("y")
            n154 = global read "Results_plotter_Global.vi" "Tolerances"() -> (w546:dbl[])
            n155 = Index Array(array=w534) -> (element #1=w526:i32, element #2=w527:i32, element #3=w525:i32)  [unwired: 3 in]
            n156 = case shown="Default" w526 {
              selector: w526 -> [_ w550]
              tunnel: w547 -> [_ w555]
              tunnel: w546 -> [_ w554]
              tunnel: [dbl[] [] ("Bin Centres") w553] -> w538
              tunnel: [w548 w552] -> w537
              tunnel: [w548 w551] -> w536
              frame -1 {
                w548 = i32[] [] ("Bin Index")
              }
              frame Default {
                n157 = Index Array(array=w555, index (col)=w550) -> (element=w558:string[])  [unwired: 1 in]
                n158 = Fract/Exp String To Number(string=w558) -> (number=w557:dbl[])  [unwired: 4 out]
                n159 = Index Array(array=w554, index=w550) -> (element=w556:dbl)
                n160 = call "Numeric_bins.vi"("Values"=w557, "Tolerance"=w556) -> ("Bin Centres"=w553:dbl[], "No of points in bins"=w552:i32[], "Bin Index"=w551:i32[])
              }
            }
            n161 = case shown="Default" w527 {
              selector: w527 -> [_ w561]
              tunnel: w547 -> [_ w566]
              tunnel: w546 -> [_ w565]
              tunnel: [dbl[] [] ("Bin Centres") w564] -> w533
              tunnel: [w559 w563] -> w532
              tunnel: [w559 w562] -> w531
              frame -1 {
                w559 = i32[] [] ("Bin Index")
              }
              frame Default {
                n162 = Index Array(array=w566, index (col)=w561) -> (element=w567:string[])  [unwired: 1 in]
                n163 = Fract/Exp String To Number(string=w567) -> (number=w568:dbl[])  [unwired: 4 out]
                n164 = Index Array(array=w565, index=w561) -> (element=w569:dbl)
                n165 = call "Numeric_bins.vi"("Values"=w568, "Tolerance"=w569) -> ("Bin Centres"=w564:dbl[], "No of points in bins"=w563:i32[], "Bin Index"=w562:i32[])
              }
            }
            n166 = case shown="Default" w525 {
              selector: w525 -> [_ w572]
              tunnel: w547 -> [_ w577]
              tunnel: w546 -> [_ w576]
              tunnel: [dbl[] [] ("Bin Centres") w575] -> w530
              tunnel: [w570 w574] -> w529
              tunnel: [w570 w573] -> w528
              frame -1 {
                w570 = i32[] [] ("No of points in bins")
              }
              frame Default {
                n167 = Index Array(array=w577, index (col)=w572) -> (element=w580:string[])  [unwired: 1 in]
                n168 = Index Array(array=w576, index=w572) -> (element=w578:dbl)
                n169 = Fract/Exp String To Number(string=w580) -> (number=w579:dbl[])  [unwired: 4 out]
                n170 = call "Numeric_bins.vi"("Values"=w579, "Tolerance"=w578) -> ("Bin Centres"=w575:dbl[], "No of points in bins"=w574:i32[], "Bin Index"=w573:i32[])
              }
            }
            n171 = Build Array (concatenate)(w537, w532, w529) -> (w545:i32[])
            n172 = Sort 1D Array(array=w545) -> (sorted array=w544:i32[])
            n173 = Reverse 1D Array(array=w544) -> (reversed array=w542:i32[])
            n174 = for {
              N: 35 -> [_]
              tunnel: w542 -> [w584] mode=indexing
              tunnel: [w585] -> w541
              tunnel: [w584] -> w540
              tunnel: w539 -> [w583]
              stop <- w585 continue-if-true
              n175 = Greater?(x=w584, y=w583) -> (0:w585:bool)
            }
            n176 = case shown="True" w541 {
              tunnel: w540 -> [_ w582]
              tunnel: [w581 w582] -> w535
              tunnel: w539 -> [w581 _]
              frame False {
              }
              frame True {
              }
            }
          }
          frame #1 {
            n177 = for {
              tunnel: w598 -> [w613] mode=indexing
              tunnel: w599 -> [w612]
              tunnel: [w611] -> w597 mode=indexing if=w609
              tunnel: w596 -> [w610] mode=indexing
              tunnel: [w610] -> w591 mode=indexing if=w609
              workers-P: _ -> [_]
              i -> [w611]
              n178 = Greater?(x=w613, y=w612) -> (0:w609:bool)
            }
            n179 = Index Array(array=w594, index=0) -> (element=w592:i32)
            n180 = Index Array(array=w593, index=w592) -> (element=w590:string)
            n181 = call "Unique_Selector_Values.vi"("Precision"=w590, "Bin Centres"=w591) -> ("Bin Strings"=w589:string[])  [unwired: 1 in, 1 out]
            n182 = for {
              tunnel: w586 -> [w605]
              tunnel: [w604] -> w588 mode=indexing
              tunnel: w597 -> [w603] mode=indexing
              workers-P: _ -> [_]
              n183 = for {
                tunnel: w605 -> [w608] mode=indexing
                tunnel: w603 -> [w607]
                tunnel: [w606] -> w604 mode=indexing
                n184 = Equal?(x=w607, y=w608) -> (x = y?=w606:bool)
              }
            }
            n185 = for {
              tunnel: w589 -> [w602] mode=indexing
              tunnel: [w600] -> w587 mode=indexing
              workers-P: _ -> [_]
              n186 = Concatenate Strings("X=" ("string"), w602) -> (w600:string)
            }
          }
          frame #2 {
            n187 = for {
              tunnel: w615 -> [w641] mode=indexing
              tunnel: w627 -> [w640]
              tunnel: [w639] -> w626 mode=indexing if=w637
              tunnel: w616 -> [w638] mode=indexing
              tunnel: [w638] -> w621 mode=indexing if=w637
              i -> [w639]
              n188 = Greater?(x=w641, y=w640) -> (0:w637:bool)
            }
            n189 = Index Array(array=w624, index=1) -> (element=w622:i32)
            n190 = Index Array(array=w623, index=w622) -> (element=w620:string)
            n191 = call "Unique_Selector_Values.vi"("Precision"=w620, "Bin Centres"=w621) -> ("Bin Strings"=w619:string[])  [unwired: 1 in, 1 out]
            n192 = for {
              tunnel: w614 -> [w633]
              tunnel: [w632] -> w618 mode=indexing
              tunnel: w626 -> [w631] mode=indexing
              n193 = for {
                tunnel: w633 -> [w636] mode=indexing
                tunnel: w631 -> [w635]
                tunnel: [w634] -> w632 mode=indexing
                n194 = Equal?(x=w635, y=w636) -> (x = y?=w634:bool)
              }
            }
            n195 = for {
              tunnel: w619 -> [w630] mode=indexing
              tunnel: [w628] -> w617 mode=indexing
              n196 = Concatenate Strings("Y=" ("string"), w630) -> (w628:string)
            }
          }
          frame #3 {
            n197 = for {
              tunnel: w643 -> [w669] mode=indexing
              tunnel: w655 -> [w668]
              tunnel: [w667] -> w654 mode=indexing if=w665
              tunnel: w642 -> [w666] mode=indexing
              tunnel: [w666] -> w649 mode=indexing if=w665
              i -> [w667]
              n198 = Greater?(x=w669, y=w668) -> (0:w665:bool)
            }
            n199 = Index Array(array=w652, index=2) -> (element=w650:i32)
            n200 = Index Array(array=w651, index=w650) -> (element=w648:string)
            n201 = call "Unique_Selector_Values.vi"("Precision"=w648, "Bin Centres"=w649) -> ("Bin Strings"=w647:string[])  [unwired: 1 in, 1 out]
            n202 = for {
              tunnel: w644 -> [w661]
              tunnel: [w660] -> w645 mode=indexing
              tunnel: w654 -> [w659] mode=indexing
              n203 = for {
                tunnel: w661 -> [w664] mode=indexing
                tunnel: w659 -> [w663]
                tunnel: [w662] -> w660 mode=indexing
                n204 = Equal?(x=w663, y=w664) -> (x = y?=w662:bool)
              }
            }
            n205 = for {
              tunnel: w647 -> [w658] mode=indexing
              tunnel: [w656] -> w646 mode=indexing
              n206 = Concatenate Strings("Z=" ("string"), w658) -> (w656:string)
            }
          }
          frame #4 {
            n207 = Build Array (concatenate)(w672, w671, w670) -> (w673:string[])
            n208 = Build Array (concatenate)(w677, w676, w675) -> (w674:bool[][])
          }
          frame #5 {
          }
        }
      }
      frame "Add Show All Rows" {
        n209 = Index Array(array=w701, index=0 ("Index")) -> (element=w699:i32)
        n210 = Initialize Array(TRUE, w699) -> (w698:bool[])
        n211 = Build Array (concatenate)(w698, w697) -> (w688:bool[][])
        n212 = Build Array (concatenate)("Show All" ("Input Element"), w696) -> (w691:string[])
        n213 = case shown="False" "notSelectors?" {
          tunnel: w691 -> [_ w715]
          tunnel: "Create Accept Array" -> [w708 w713]
          tunnel: [w708 w711] -> w689
          tunnel: w687 -> [_ w709]
          frame False {
          }
          frame True {
            n214 = Array Size(array=w715) -> (size(s)=w714:i32)
            n215 = Greater?(x=w714, y=w709) -> (0:w710:bool)
            n216 = Select(t=w713, s=w710, f="Add NOT Selectors") -> (s? t:f=w711:string)
          }
        }
      }
      frame "Add NOT Selectors" {
        n217 = Increment(x=w727) -> (x+1=w726:i32)
        n218 = Array Subset(array=w723, index (row)=w726) -> (w725:bool[][])  [unwired: 3 in]
        n219 = Array Subset(array=w719, index=w726) -> (w721:string[])  [unwired: 1 in]
        n220 = Not(x=w725) -> (.not. x?=w724:bool[][])
        n221 = for {
          tunnel: w721 -> [w736] mode=indexing
          tunnel: [w735] -> w720 mode=indexing
          workers-P: _ -> [_]
          n222 = Concatenate Strings("NOT " ("string"), w736) -> (w735:string)
        }
        n223 = Build Array (concatenate)(w723, w724) -> (w722:bool[][])
        n224 = Build Array (concatenate)(w719, w720) -> (w718:string[])
      }
      frame "Create Accept Array" {
        n225 = for {
          tunnel: w744 -> [w770] mode=indexing
          tunnel: w740 -> [w769]
          shift-right: [w766] -> w748
          shift-left: _ -> [w767]
          tunnel: w743 -> [w765]
          tunnel: [w763] -> w738 mode=indexing
          i -> [w768]
          n226 = Index Array(array=w769, index (row)=w770) -> (element=w763:bool[])  [unwired: 1 in]
          n227 = And(x=w765, y=w763) -> (x .and. y?=w764:bool[])
          n228 = case shown="1, Default" w768 {
            tunnel: w767 -> [_ w774]
            tunnel: [w771 w773] -> w766
            tunnel: w764 -> [w771 w772]
            frame 0 {
            }
            frame 1, Default {
              n229 = Or(x=w772, y=w774) -> (x .or. y?=w773:bool[])
            }
          }
        }
        "Accept array" <- w738
        n230 = for {
          tunnel: w749 -> [w759]
          tunnel: [w757] -> w746 mode=indexing
          tunnel: w747 -> [w756] mode=indexing
          tunnel: w748 -> [w755]
          workers-P: _ -> [_]
          i -> [w760]
          n231 = Equal?(x=w759, y=w760) -> (x = y?=w758:bool)
          n232 = case shown="False" w758 {
            tunnel: [w761 w762] -> w757
            tunnel: w756 -> [w761 _]
            tunnel: w755 -> [_ w762]
            frame False {
            }
            frame True {
            }
          }
        }
      }
      frame "Add Number of hits" {
        n233 = for {
          tunnel: w796 -> [w827]
          tunnel: w792 -> [w825] mode=indexing
          shift-right: [w823] -> w786
          shift-left: w794 -> [w824]
          i -> [w822]
          n234 = Equal?(x=w827, y=w822) -> (x = y?=w826:bool)
          n235 = case shown="False" w826 {
            tunnel: w825 -> [w830 _]
            tunnel: w824 -> [w829 w831]
            tunnel: [w828 w831] -> w823
            frame False {
              n236 = And(x=w830, y=w829) -> (x .and. y?=w828:bool[])
            }
            frame True {
            }
          }
        }
        n237 = Array Size(array=w784) -> (size(s)=w783:i32[])
        n238 = Index Array(array=w783, index=0) -> (element=w781:i32)
        n239 = Multiply(x=3, y=w778) -> (x*y=w779:i32)
        n240 = Less?(x=w781, y=w779) -> (x < y?=w780:bool)
        n241 = for {
          tunnel: w786 -> [w809]
          tunnel: w784 -> [w808] mode=indexing
          tunnel: w787 -> [w814] mode=indexing
          tunnel: [w813] -> w790 mode=indexing
          tunnel: [w805] -> w789 mode=indexing
          shift-right: [w806] -> _
          shift-left: 0 -> [w807]
          tunnel: w780 -> [w802]
          tunnel: w776 -> [w800]
          n242 = And(x=w809, y=w808) -> (x .and. y?=w810:bool[])
          n243 = Boolean To (0,1)(Boolean=w810) -> (0, 1=w811:i16[])
          n244 = To Long Integer(number=w811) -> (32bit integer=w801:i32[])
          n245 = Add Array Elements(numeric array=w801) -> (sum=w812:i32)
          n246 = Greater Than 0?(x=w812) -> (x > 0?=w803:bool)
          n247 = Format Into String(format string=" (%d)" ("Format String"), initial string=w814, w812) -> (resulting string=w813:string)  [unwired: 1 in, 1 out]
          n248 = Or(x=w803, y=w802) -> (x .or. y?=w804:bool)
          n249 = case shown="True" w804 {
            tunnel: w807 -> [w816 w820]
            tunnel: [w816 w821] -> w806
            tunnel: [FALSE w819] -> w805
            tunnel: w800 -> [_ w818]
            frame False {
            }
            frame True {
              n250 = Increment(x=w820) -> (x+1=w821:i32)
              n251 = Less?(x=w820, y=w818) -> (x < y?=w819:bool)
            }
          }
        }
      }
      frame "Relocate Selector?" {
        n252 = Index Array(array=w843, index=w835) -> (element=w844:T1)
        n253 = Unbundle By Name(w844) -> ("Bin Names"=w842:string[])
        n254 = Array Size(array=w842) -> (size(s)=w841:i32)
        n255 = Greater Than 0?(x=w841) -> (x > 0?=w839:bool)
        n256 = Select(t="Relocate Selector", s=w839, f="Stop invalid selections") -> (s? t:f=w837:string)
      }
      frame "Relocate Selector" {
        n257 = Index Array(array=w855, index=w863) -> (element=w860:T1)
        n258 = Unbundle By Name(w860) -> ("Bin Names"=w861:string[])
        n259 = for {
          tunnel: w864 -> [w870] mode=indexing
          tunnel: [w869] -> w858 mode=indexing
          n260 = Match Pattern(string=w870, regular expression=" (") -> (before substring=w869:string)  [unwired: 4 out]
        }
        n261 = for {
          tunnel: w857 -> [w872] mode=indexing
          tunnel: w861 -> [w878]
          tunnel: w858 -> [w876]
          shift-right: [w873] -> w852
          shift-left: i32[] [] -> [w874]
          n262 = Index Array(array=w878, index=w872) -> (element=w875:string)
          n263 = Search 1D Array(1D array=w876, element=w875) -> (index of element=w877:i32)  [unwired: 1 out]
          n264 = case shown="0, Default" w877 {
            selector: w877 -> [w879 _]
            tunnel: w874 -> [w881 w882]
            tunnel: [w880 w882] -> w873
            frame 0, Default {
              n265 = Build Array (concatenate)(w881, w879) -> (w880:i32[])
            }
            frame -1 {
            }
          }
        }
      }
      frame "Stop invalid selections" {
        n266 = Array Size(array=w888) -> (size(s)=w889:i32)
        n267 = case shown="2, Default" w889 {
          tunnel: [i32[] [0] w898 w899] -> w884
          tunnel: w888 -> [_ w898 w901]
          frame 0 {
          }
          frame 1 {
          }
          frame 2, Default {
            n268 = for {
              tunnel: w901 -> [w902] mode=indexing
              shift-right: [w903] -> w899
              shift-left: i32[] [] -> [w904]
              n269 = Equal To 0?(x=w902) -> (x = 0?=w905:bool)
              n270 = case shown="False" w905 {
                tunnel: w904 -> [w907 w909]
                tunnel: [w906 w909] -> w903
                tunnel: w902 -> [w908 _]
                frame False {
                  n271 = Build Array (concatenate)(w907, w908) -> (w906:i32[])
                }
                frame True {
                }
              }
            }
          }
        }
      }
      frame "Update shift Register" {
        n272 = for {
          tunnel: w917 -> [w959] mode=indexing
          tunnel: [w958] -> w923 mode=indexing
          workers-P: _ -> [_]
          n273 = Match Pattern(string=w959, regular expression=" (") -> (before substring=w958:string)  [unwired: 4 out]
        }
        n274 = Index Array(array=w931, index=w932) -> (element=w926:T1)
        n275 = for {
          shift-right: [w943] -> w914
          shift-left: string[] [] -> [w946]
          tunnel: w918 -> [w949] mode=indexing
          shift-right: [w944] -> w913
          shift-left: i32[] [] -> [w945]
          tunnel: w917 -> [w947] mode=indexing
          i -> [w948]
          n276 = case shown="True" w949 {
            tunnel: w948 -> [_ w957]
            tunnel: w947 -> [_ w956]
            tunnel: w946 -> [w951 w955]
            tunnel: w945 -> [w950 w954]
            tunnel: [w950 w953] -> w944
            tunnel: [w951 w952] -> w943
            frame False {
            }
            frame True {
              n277 = Build Array (concatenate)(w955, w956) -> (w952:string[])
              n278 = Build Array (concatenate)(w954, w957) -> (w953:i32[])
            }
          }
        }
        n279 = Index Array(array=w929, index=0 ("Index")) -> (element=w922:i32)
        n280 = for {
          tunnel: w913 -> [w942]
          tunnel: w912 -> [w941] mode=indexing
          tunnel: [w937] -> w911 mode=indexing
          workers-P: _ -> [_]
          n281 = Search 1D Array(1D array=w942, element=w941) -> (index of element=w938:i32)  [unwired: 1 out]
          n282 = In Range and Coerce(upper limit=65000, x=w938, lower limit=0) -> (coerced(x)=w937:i32)  [unwired: 1 out]
        }
        n283 = Bundle By Name(cluster=w926, "Bin Matches"=w925, "Channel to Filter On"=w924, "Bin Names"=w923, "Number of Rows"=w922, "Tolerance"=w920, "Filter Bins"=w911, "Indicies for all bins"=w913) -> (w921:T1)
        n284 = Replace Array Subset(array=w931, new element=w921, index=w932) -> (w930:T2)
      }
    }
  }
  "Filter Bins Out" <- w10
  n285 = Array Size(array=w6) -> (size(s)=w5:i32)
  n286 = Index Array(array=w6, index=w7) -> (element=w3:string)
  n287 = Decrement(x=w5) -> (x-1=w4:i32)
  n288 = Format Into String(format string=" -- # of Bins (%d)", initial string=w3, w4) -> (resulting string=w1:string)  [unwired: 1 in, 1 out]
  n289 = Replace Array Subset(array=w6, new element=w1, index=w7) -> (→"Bin Names":string[])
